vi "Warp Affine.vi"   [LabVIEW 2020, in "image.lvlib"]
doc: "Warp the Source Image according to the given 2x3 Affine Matrix."
uses:
  image.lvlib
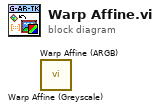
[diagram p0: block diagram]
diagram:
  n1 = call "Warp Affine (Greyscale).vi"() -> ()  [unwired: 10 in, 2 out]
  n2 = call "Warp Affine (ARGB).vi"() -> ()  [unwired: 10 in, 2 out]
